vi "Delete Sensor.vi"(0 "Sensors":T2[](array[typedef]) {"Max Error % of Reading" format="%.2f"; "Max Stability Error" format="%.2f"; "Max Mean Squared Error" format="%.2f"; "Max Error % of Full Scale" format="%.2f"; "Coefficients" format="%.2f"; "Voltage List" format="%.2f"; "EGU List" format="%.2f"; "EGU Range"."Low Limit" format="%.2f"; "EGU Range"."High Limit" format="%.2f"; "Voltage Range"."Low Limit" format="%.2f"; "Voltage Range"."High Limit" format="%.2f"; "Last Cal Info"."Last Calibration Date" format="%.2f"}) -> (4 "Sensors out":T1(array[cluster]))   [LabVIEW 2023]
uses:
  Type Defs and Controls/Sensor.ctl
panel:
  in  "Cancel Button":bool
  in  "Delete":bool
  in  "Available Sensors":i32(listbox)
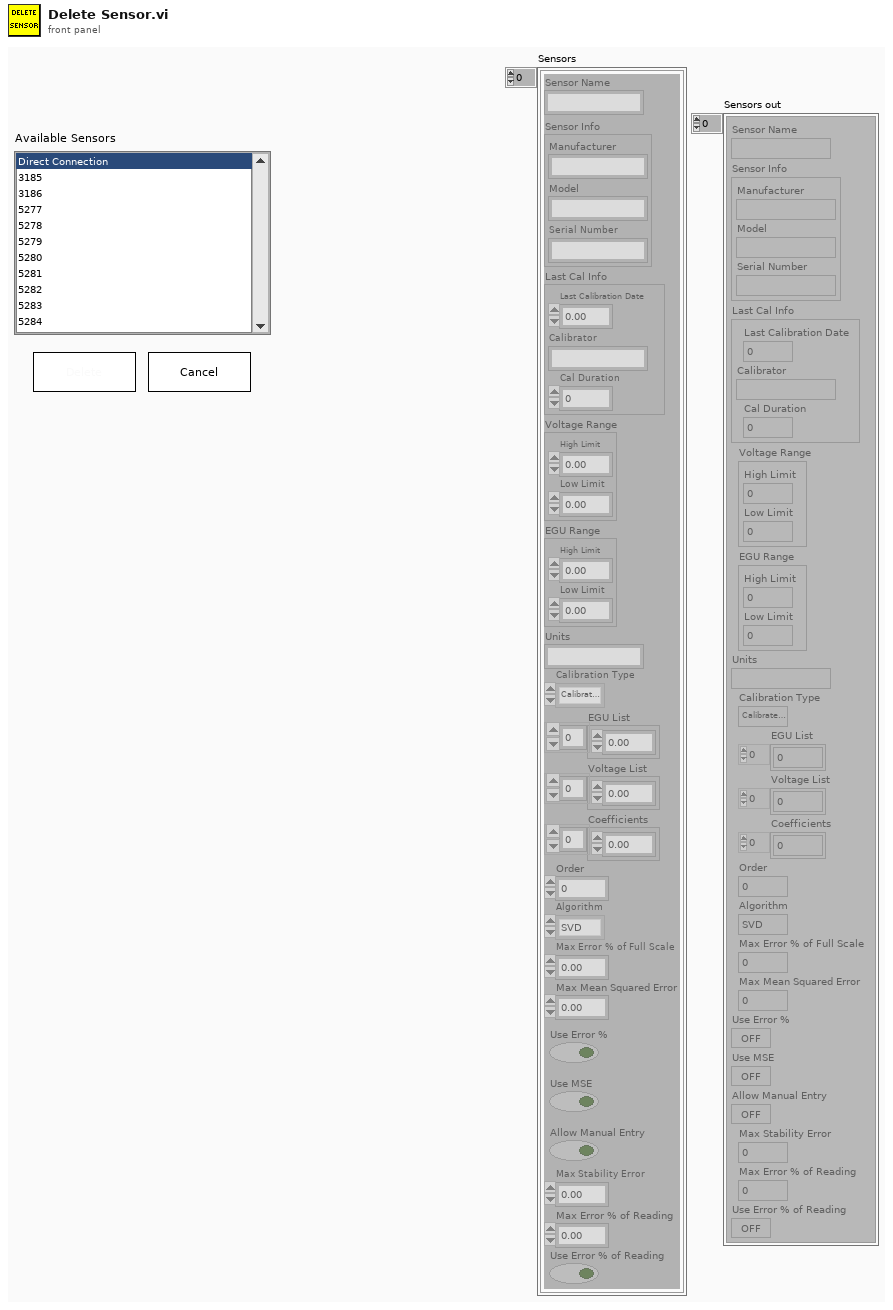
[diagram p1: front panel]
types:
  T1 = cluster{"Sensor Name":string, "Sensor Info":cluster{"Manufacturer":string, "Model":string, "Serial Number":string}, "Last Cal Info":cluster{"Last Calibration Date":dbl, "Calibrator":string, "Cal Duration":i32}, "Voltage Range":cluster{"High Limit":dbl, "Low Limit":dbl}, "EGU Range":cluster{"High Limit":dbl, "Low Limit":dbl}, "Units":string, "Calibration Type":enum16{"Calibrate Analog", "Compare Analog Calibration"}, "EGU List":dbl[], "Voltage List":dbl[], "Coefficients":dbl[], "Order":i32, "Algorithm":enum32{"SVD", "Givens", "Givens2", "Householder", "LU Decomposition", "Cholesky"}, "Max Error % of Full Scale":dbl, "Max Mean Squared Error":dbl, "Use Error %":bool, "Use MSE":bool, "Allow Manual Entry":bool, "Max Stability Error":dbl, "Max Error % of Reading":dbl, "Use Error % of Reading":bool}[]
  T2 = typedef "Sensor.ctl" = cluster{"Sensor Name":string, "Sensor Info":cluster{"Manufacturer":string, "Model":string, "Serial Number":string}, "Last Cal Info":cluster{"Last Calibration Date":dbl, "Calibrator":string, "Cal Duration":i32}, "Voltage Range":cluster{"High Limit":dbl, "Low Limit":dbl}, "EGU Range":cluster{"High Limit":dbl, "Low Limit":dbl}, "Units":string, "Calibration Type":enum16{"Calibrate Analog", "Compare Analog Calibration"}, "EGU List":dbl[], "Voltage List":dbl[], "Coefficients":dbl[], "Order":i32, "Algorithm":enum32{"SVD", "Givens", "Givens2", "Householder", "LU Decomposition", "Cholesky"}, "Max Error % of Full Scale":dbl, "Max Mean Squared Error":dbl, "Use Error %":bool, "Use MSE":bool, "Allow Manual Entry":bool, "Max Stability Error":dbl, "Max Error % of Reading":dbl, "Use Error % of Reading":bool}
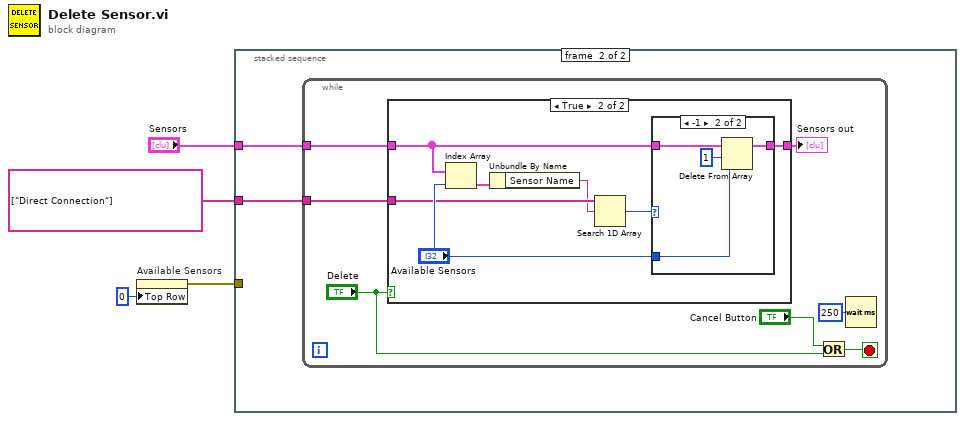
[diagram p0: block diagram]
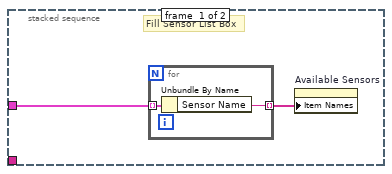
[diagram p2: hidden frame]
diagram:
  n1 = property on="Available Sensors" class="LstBox (strict)"("Top Row"=0) -> (error out=w1:errorcluster)  [unwired: 2 in, 1 out]
  n2 = stacked-sequence {
    tunnel: "Sensors" -> [w5 w10]
    tunnel: string[] ["Direct Connection"] -> [_ w9]
    tunnel: w1 -> [_ _]
    frame #0 {
      # "Fill Sensor List Box"
      n3 = for {
        tunnel: w5 -> [w8] mode=indexing
        tunnel: [w7] -> w6 mode=indexing
        n4 = Unbundle By Name(w8) -> ("Sensor Name"=w7:string)
      }
      n5 = property on="Available Sensors" class="LstBox (strict)"("Item Names"=w6) -> ()  [unwired: 2 in, 2 out]
    }
    frame #1 {
      n6 = while {
        tunnel: w10 -> [w14]
        tunnel: w9 -> [w11]
        stop <- w17 stop-if-true
        n7 = case shown="True" "Delete" {
          tunnel: w14 -> [w18 w24]
          tunnel: [w18 w25] -> w13
          tunnel: w11 -> [_ w22]
          frame False {
          }
          frame True {
            n8 = Index Array(array=w24, index="Available Sensors") -> (element=w21:T2)
            n9 = Unbundle By Name(w21) -> ("Sensor Name"=w20:string)
            n10 = Search 1D Array(1D array=w22, element=w20) -> (index of element=w19:i32)  [unwired: 1 in]
            n11 = case shown="-1" w19 {
              tunnel: [w26 w30] -> w25
              tunnel: w24 -> [w26 w28]
              tunnel: "Available Sensors" -> [_ w27]
              frame Default {
              }
              frame -1 {
                n12 = Delete From Array(array=w28, length=1, index=w27) -> (array with subset deleted=w30:T2[])  [unwired: 1 out]
              }
            }
          }
        }
        "Sensors out" <- w13
        n13 = Or(x="Cancel Button", y="Delete") -> (x .or. y?=w17:bool)
        n14 = Wait (ms)(milliseconds to wait=u32 250) -> ()  [unwired: 1 out]
      }
    }
  }
